vi "Controller - Log File.vi"(7 "filename":string="status_log.txt", 8 "error in":errorcluster, 11 "Status":string) -> (0 "error out":errorcluster)   [LabVIEW 2017]
doc: "This SubVI create new or replace existing text file (Status_log.txt) data \nabout actual status and current timestamp."
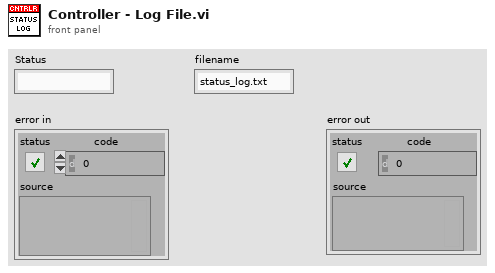
[diagram p1: front panel]
types:
  T1 = enum16{"open", "replace", "create", "open or create", "replace or create", "replace or create with confirmation"}
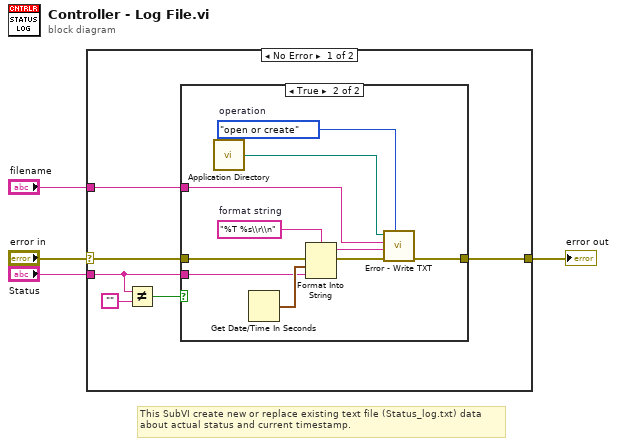
[diagram p0: block diagram]
diagram:
  # "This SubVI create new or replace existing text file (Status_log.txt) data \nabout actual status and current timestamp."
  n1 = case shown="No Error" "error in" {
    selector: "error in" -> [w10 w22]
    tunnel: [w9 w22] -> w4
    tunnel: "Status" -> [w6 _]
    tunnel: "filename" -> [w5 _]
    frame No Error {
      n2 = Not Equal?(x=w6, y="") -> (x != y?=w7:bool)
      n3 = case shown="True" w7 {
        tunnel: w10 -> [w11 w16]
        tunnel: [w11 w14] -> w9
        tunnel: w6 -> [_ w13]
        tunnel: w5 -> [_ w12]
        frame False {
        }
        frame True {
          w15 = T1."open or create"  # operation
          w21 = "%T %s\\r\\n"  # format string
          n4 = call <vilib>:"Application Directory.vi"() -> ("Application Directory"=w19:path)
          n5 = Get Date/Time In Seconds() -> (seconds since 1Jan1904=w20:timestamp)
          n6 = Format Into String(format string=w21, error in=w16, w20, w13) -> (resulting string=w17:string, error out=w18:errorcluster)  [unwired: 1 in]
          n7 = call "Error - Write TXT.vi"("operation"=w15, "error in"=w18, "text"=w17, "filename.txt"=w12, "base path"=w19) -> ("error out"=w14:errorcluster)  [unwired: 6 in]
        }
      }
    }
    frame Error {
      # "If NO Error occurred"
    }
  }
  "error out" <- w4
